vi "Find Family.vi"(8 "error in (no error)":errorcluster, 10 "Panel":string) -> (0 "error out":errorcluster, 1 "Children":string[](array[string]), 2 "Ancestors":string[](array[string]))   [LabVIEW 2019]
uses:
  <vilib>/MGI/Panel Manager/Panel/Panel Registry/Panel Registry.lvclass
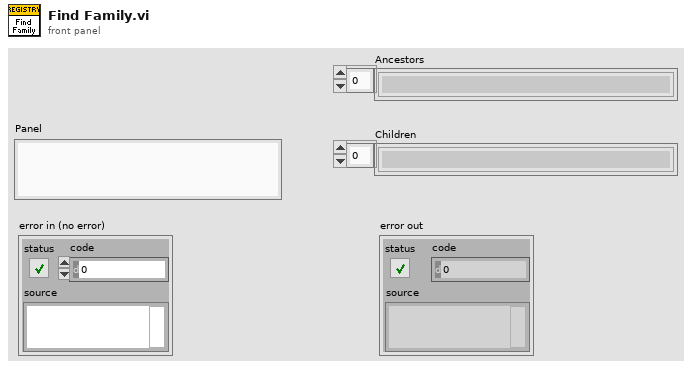
[diagram p1: front panel]
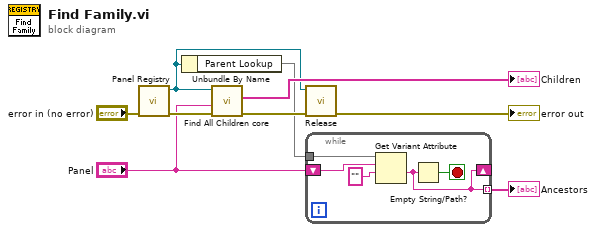
[diagram p0: block diagram]
diagram:
  n1 = call <vilib>:"Panel Registry.vi"("error in (no error)"="error in (no error)") -> ("error out"=w9:errorcluster, "Panel Registry out"=w4:refnum<class "Panel Registry.lvclass">)  [unwired: 9 in]
  n2 = Unbundle By Name(w4) -> ("Parent Lookup"=w1)
  n3 = call <vilib>:"Find All Children core.vi"("error in (no error)"=w9, "Panel"="Panel", "Panel Registry in"=w4) -> ("error out"=w8:errorcluster, "All Children"=→"Children":string[])  [unwired: 7 in]
  n4 = call <vilib>:"Release.vi"("error in (no error)"=w8, "Panel Registry in"=w4) -> ("error out"=→"error out":errorcluster)  [unwired: 9 in]
  n5 = while {
    shift-right: [w10] -> _
    shift-left: "Panel" -> [w12]
    tunnel: [w10] -> w3 mode=indexing
    tunnel: w1 -> [w13]
    stop <- w14 stop-if-true
    n6 = Get Variant Attribute(Variant=w13, name=w12, default value (empty Variant)="" ("VI")) -> (value=w10:string)  [unwired: 1 in, 3 out]
    n7 = Empty String/Path?(string/path=w10) -> (empty?=w14:bool)
  }
  "Ancestors" <- w3
